vi "Load Async.vi"(8 "error in (no error)":errorcluster, 10 "Path":path, 11 "Channel in":refnum<data-value>) -> (0 "error out":errorcluster, 3 "Channel out":refnum<data-value>)   [LabVIEW 2020, in "G-Audio.lvlib" / "Channel.lvclass"]
uses:
  Channel.lvclass
  G-Audio.lvlib
  Channel State.ctl
  Mixer/Mixer Audio Data Type.ctl
  Mixer/Mixer.lvclass
  Audio Files/Polymorphic VIs/Open Audio File Read (Path).vi
  Audio Files/Polymorphic VIs/Get Audio File Info (Path).vi
  88edfe70-fc9c-4621-9b1b-9ed93909f707.vi
  8ac861a4-dc9e-40dd-a8dd-4f0d9c8cf1a7.vi
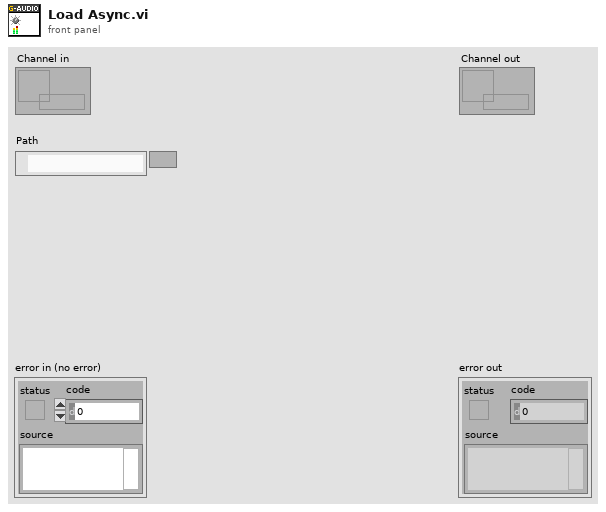
[diagram p1: front panel]
types:
  T1 = typedef "G-Audio.lvlib/Channel.lvclass/Channel State.ctl" = enum16{"Empty", "Loading", "Stopped", "Paused", "Playing", "Retrigger"}
  T2 = typedef "G-Audio.lvlib/Mixer.lvclass/Mixer Audio Data Type.ctl" = i16[][]
  T3 = typedef "G-Audio.lvlib/Audio File Info.ctl" = cluster{"Sample Rate (Hz)":u32, "Channels":u32, "Bit Depth":u32}
  T4 = typedef "G-Audio.lvlib/Audio File Refnum.ctl" = refnum<file>
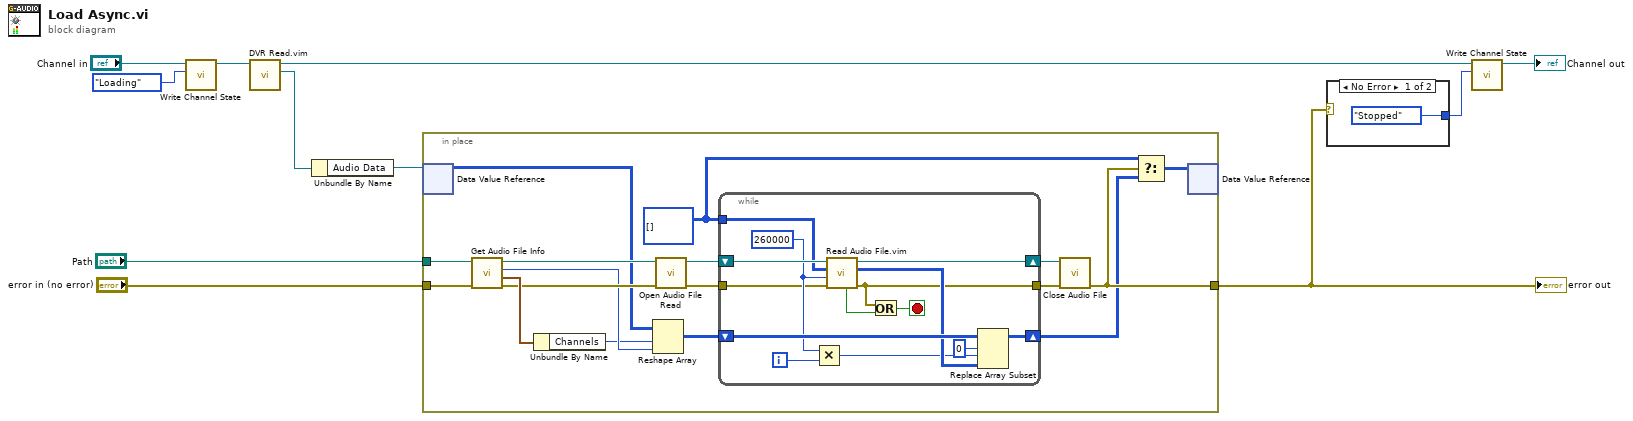
[diagram p0: block diagram]
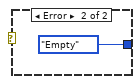
[diagram p2: hidden frame]
diagram:
  n1 = call "Write Channel State.vi"("State"=Channel_State."Loading", "Channel in"="Channel in") -> ("Channel out"=w2:refnum<data-value>)  [unwired: 8 in, 1 out]
  n2 = call "DVR Read.vim"("DVR In"=w2) -> ("Data"=w3:refnum<class "Channel.lvclass">, "DVR Out"=w1:refnum<data-value>)  [unwired: 9 in]
  n3 = Unbundle By Name(w3) -> ("Audio Data"=w4:refnum<data-value>)
  n4 = in-place {
    in-place-border: "Path" -> [w21]
    in-place-border: "error in (no error)" -> [w20]
    in-place-border: [w15] -> w7
    w12 = T2 [] ("Audio Data Type")
    n5 = in-place-dvr #1(w4) -> (w19:T2)  [unwired: 1 out]
    n6 = call-poly "Get Audio File Info.vi"("error in (no error)"=w20, "Path In"=w21) -> ("error out"=w26:errorcluster, "Audio File Info"=w28:T3, "PCM Frame Length"=w18:u64, "Path Out"=w27:path)  [unwired: 5 in, 1 out]
    n7 = Unbundle By Name(w28) -> ("Channels"=w17:u32)
    n8 = Reshape Array(w19, w17, w18) -> (w16:T2)
    n9 = call-poly "Open Audio File Read.vi"("error in (no error)"=w26, "Path"=w27) -> ("error out"=w22:errorcluster, "Audio File Refnum"=w25:T4)  [unwired: 8 in]
    n10 = while {
      shift-right: [w34] -> w14
      shift-left: w16 -> [w40]
      shift-right: [w33] -> w24
      shift-left: w25 -> [w42]
      tunnel: w12 -> [w41]
      tunnel: [w29] -> w23
      tunnel: w22 -> [w32]
      i -> [w37]
      stop <- w30 stop-if-true
      w36 = u64 260000 ("Frames To Read")
      n11 = Multiply(x=w36, y=w37) -> (x*y=w35:u64)
      n12 = call "Read Audio File.vim"("error in (no error)"=w32, "Frames To Read"=w36, "Data Format"=w41, "Audio File Refnum In"=w42) -> ("error out"=w29:errorcluster, "Audio Data"=w39:T2, "Audio File Refnum Out"=w33:T4, "End of File?"=w31:bool)  [unwired: 3 in, 1 out]
      n13 = Or(x=w29, y=w31) -> (x .or. y?=w30:bool)
      n14 = Replace Array Subset(array=w40, new element=w39, index (row)=0 ("disabled index (row)"), index (col)=w35) -> (w34:T2)
    }
    n15 = call "Close Audio File.vi"("error in (no error)"=w23, "Audio File Refnum In"=w24) -> ("error out"=w15:errorcluster)  [unwired: 9 in]
    n16 = Select(t=w12, s=w15, f=w14) -> (s? t:f=w13:T2)
    n17 = in-place-dvr #1(w13) -> ()  [unwired: 2 out]
  }
  "error out" <- w7
  n18 = case shown="No Error" w7 {
    tunnel: [Channel_State."Stopped" ("State") Channel_State."Empty" ("State")] -> w11
    frame No Error {
    }
    frame Error {
    }
  }
  n19 = call "Write Channel State.vi"("State"=w11, "Channel in"=w1) -> ("Channel out"=→"Channel out":refnum<data-value>)  [unwired: 8 in, 1 out]
